vi "muParser Multi Test.vi"() -> ()   [LabVIEW 2015]
uses:
  muExpr/muExpr.lvclass/muExpr.ctl
  muExpr/Set Variable Value.vi
  muExpr/Eval.vi
  mupLib/mupSetVarValue.vi
  mupLib/mupEval.vi
  mupLib/mupCheckError.vi
  <vilib>/Utility/error.llb/Error Cluster From Error Code.vi
  muExpr/muExpr.lvclass
panel:
  out "Instance":i32
  out "Result":dbl
  out "error out":errorcluster
  in  "Instances":i32
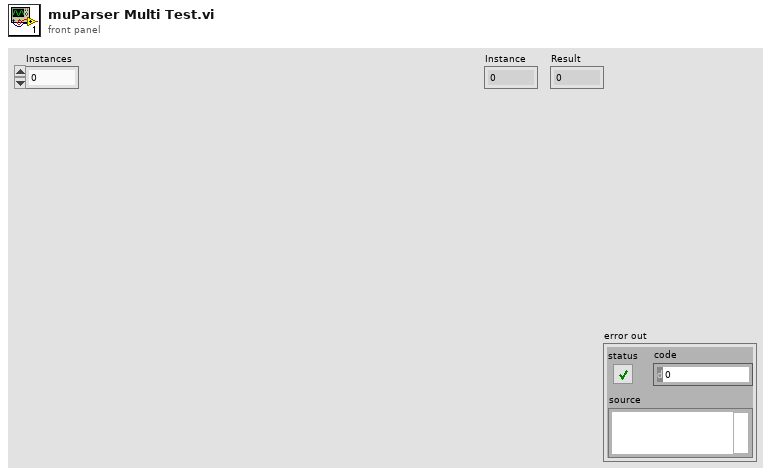
[diagram p1: front panel]
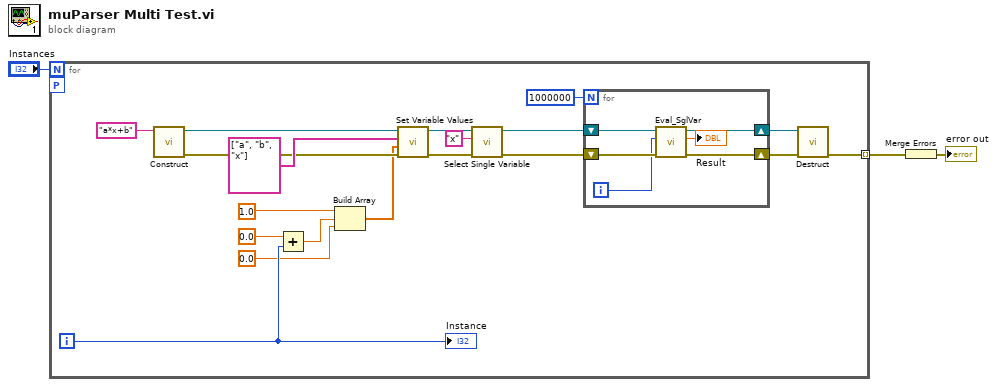
[diagram p0: block diagram]
diagram:
  n1 = for {
    N: "Instances" -> [_]
    tunnel: [w4] -> w1 mode=indexing
    workers-P: _ -> [_]
    i -> [w17]
    n2 = call "Construct.vi"("Expression"="a*x+b") -> ("error out"=w19:errorcluster, "muExpr out"=w21:refnum<class "muExpr.lvclass">)  [unwired: 8 in, 1 out]
    n3 = Add(x=0.0, y=w17) -> (x+y=w15:dbl)
    n4 = Build Array(1.0, w15, 0.0) -> (w13:dbl[])
    n5 = call "Set Variable Values.vi"("error in (no error)"=w19, "varValues"=w13, "varNames"=string[] ["a", "b", "x"], "muExpr in"=w21) -> ("error out"=w11:errorcluster, "muExpr out"=w12:refnum<class "muExpr.lvclass">)  [unwired: 6 in]
    n6 = call "Select Single Variable.vi"("error in (no error)"=w11, "varName"="x", "muExpr in"=w12) -> ("error out"=w7:errorcluster, "muExpr out"=w8:refnum<class "muExpr.lvclass">)  [unwired: 7 in]
    n7 = for {
      N: 1000000 -> [_]
      shift-right: [w25] -> w6
      shift-left: w8 -> [w28]
      shift-right: [w26] -> w5
      shift-left: w7 -> [w27]
      i -> [w24]
      n8 = call "Eval_SglVar.vi"("error in (no error)"=w27, "varValue"=w24, "muExpr in"=w28) -> ("error out"=w26:errorcluster, "Result"=→"Result":dbl, "muExpr out"=w25:refnum<class "muExpr.lvclass">)  [unwired: 6 in]
    }
    n9 = call "Destruct.vi"("error in (no error)"=w5, "muExpr in"=w6) -> ("error out"=w4:errorcluster)  [unwired: 9 in]
    "Instance" <- w17
  }
  n10 = Merge Errors(w1) -> (→"error out":errorcluster)
